vi "Get Server State UE.vi"(8 "error in":errorcluster, 11 "Template Server in":refnum<class "Servicer.lvclass">) -> (0 "error out":errorcluster, 2 "Server Internal State UE":refnum<user-event>, 3 "Template Server out":refnum<class "Servicer.lvclass">)   [LabVIEW 2019, in "gRPC-servicer.lvlib" / "Servicer.lvclass"]
uses:
  Servicer.lvclass
  Server State Data.ctl
  Servicer.lvclass/Servicer.ctl
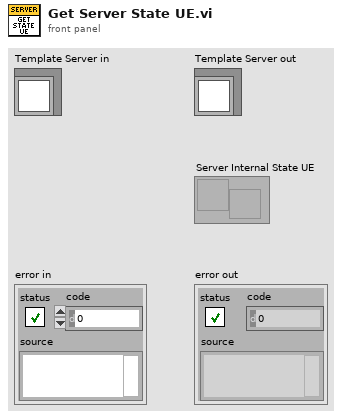
[diagram p1: front panel]
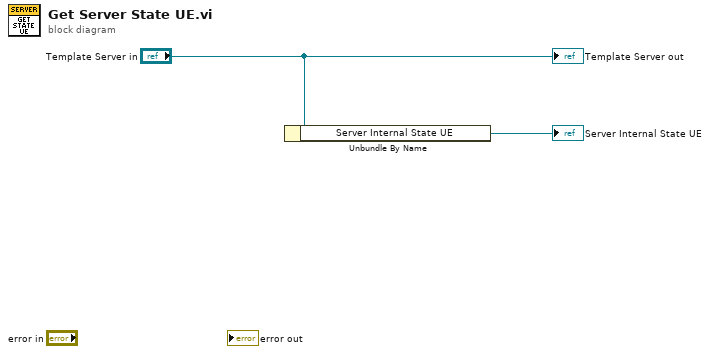
[diagram p0: block diagram]
diagram:
  n1 = Unbundle By Name("Template Server in") -> ("Server Internal State UE"=→"Server Internal State UE":refnum<user-event>)
  "Template Server out" <- "Template Server in"
